vi "armAngleToEncoderCounts.vi"() -> ()   [LabVIEW 2020]
panel:
  out "encoderCount":dbl
  in  "armAngle":dbl
  in  "b":dbl=-120.0
  in  "m":dbl=0.5
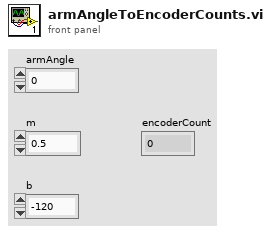
[diagram p1: front panel]
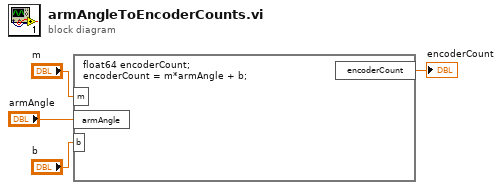
[diagram p0: block diagram]
diagram:
  n1 = formula code="float64 encoderCount;\nencoderCount = m*armAngle + b;"("m"="m", "armAngle"="armAngle", "b"="b") -> ("encoderCount"=→"encoderCount":dbl)
